vi "MoveAbsMultiple.vi"(5 "positions":dbl[](array[numeric]), 7 "speeds":dbl[](array[numeric]) min=0.0, 8 "error in (no error)":errorcluster, 9 "taskId":i32(ring) items=["TLibrary", "T01", "T02", "T03", "T04", "T05", "T06", "T07", "T08", "T09", "T10", "T11", "T12", "T13", "T14", "T15", "T16", "T17", "T18", "T19", "T20", "T21", "T22", "T23", "T24", "T25", "T26", "T27", "T28", "T29", "T30", "T31"], 10 "axis names":string[](array[string]), 11 "controller in":refnum<k24>) -> (0 "error out":errorcluster, 3 "controller out":refnum<k24>)   [LabVIEW 2020, in "Aerotech VIs.lvlib"]
uses:
  Aerotech VIs.lvlib
  C:/Program Files (x86)/Aerotech/A3200/LabVIEW/2010/Bin/Aerotech.A3200.dll
  Program Files (x86)/Aerotech/A3200/LabVIEW/2010/Bin/Aerotech.A3200.dll
  C:/Program Files (x86)/Aerotech/A3200/LabVIEW/2010/Bin/Aerotech.A3200.LabVIEW.dll
  Program Files (x86)/Aerotech/A3200/LabVIEW/2010/Bin/Aerotech.A3200.LabVIEW.dll
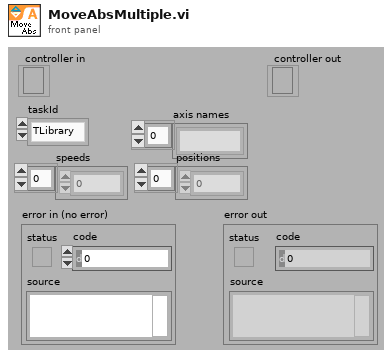
[diagram p1: front panel]
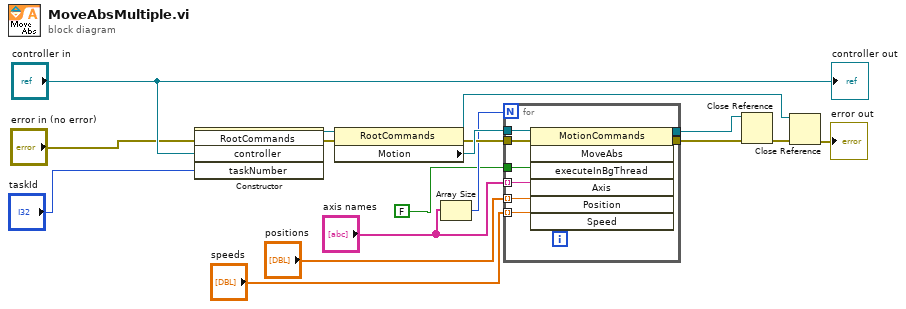
[diagram p0: block diagram]
diagram:
  n1 = constructor class="RootCommands"(error in="error in (no error)", "controller"="controller in", "taskNumber"="taskId") -> (reference out=w12:refnum<k24>, error out=w11:errorcluster)  [unwired: 2 in, 3 out]
  n2 = property class="RootCommands"(reference=w12, error in=w11) -> (reference out=w7:refnum<k24>, error out=w13:errorcluster, "Motion"=w14:refnum<k24>)
  n3 = Array Size(array="axis names") -> (size(s)=w5:i32)
  n4 = for {
    N: w5 -> [_]
    tunnel: FALSE ("return immediately") -> [w25]
    tunnel: w14 -> [w24]
    tunnel: w13 -> [w23]
    tunnel: [w22] -> w10
    tunnel: [w21] -> w9
    tunnel: "axis names" -> [w20] mode=indexing
    tunnel: "positions" -> [w19] mode=indexing
    tunnel: "speeds" -> [w18] mode=indexing
    n5 = invoke class="MotionCommands" method="MoveAbs"(reference=w24, error in=w23, "executeInBgThread"=w25, "Axis"=w20, "Position"=w19, "Speed"=w18) -> (reference out=w21:refnum<k24>, error out=w22:errorcluster)  [unwired: 1 in, 5 out]
  }
  n6 = Close Reference(reference=w9, error in (no error)=w10) -> (error out=w8:errorcluster)
  n7 = Close Reference(reference=w7, error in (no error)=w8) -> (error out=→"error out":errorcluster)
  "controller out" <- "controller in"
